vi "SNTP Light RT Driver VI_SNTP Part.vi"(7 "Configuration":T1={"Server IP Address"="206.246.122.250", "UDP Port"=123, "Synchronization Interval"=60.0, "Synchronization Threshold"=0.01, "Debug Output Strings"=TRUE, "Maximum Offset To Apply"=0.0}, 8 "error in (no error)":errorcluster, 9 "Inputs In":dbl[](array[numeric]), 11 "Outputs In":dbl[](array[numeric])) -> (0 "error out":errorcluster, 3 "Outputs Out":dbl[](array[numeric]))   [LabVIEW 2013, in "SNTP Light Custom Device Engine.lvlib"]
uses:
  SNTP Light Custom Device Engine.lvlib
  RT_Configuration_Data.ctl
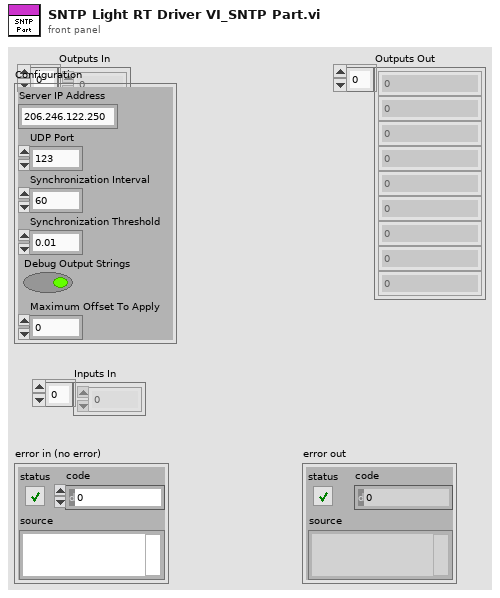
[diagram p1: front panel]
types:
  T1 = typedef "SNTP Light Custom Device Engine.lvlib/RT_Configuration_Data.ctl" = cluster{"Server IP Address":string, "UDP Port":u16, "Synchronization Interval":dbl, "Synchronization Threshold":dbl, "Debug Output Strings":bool, "Maximum Offset To Apply":dbl}
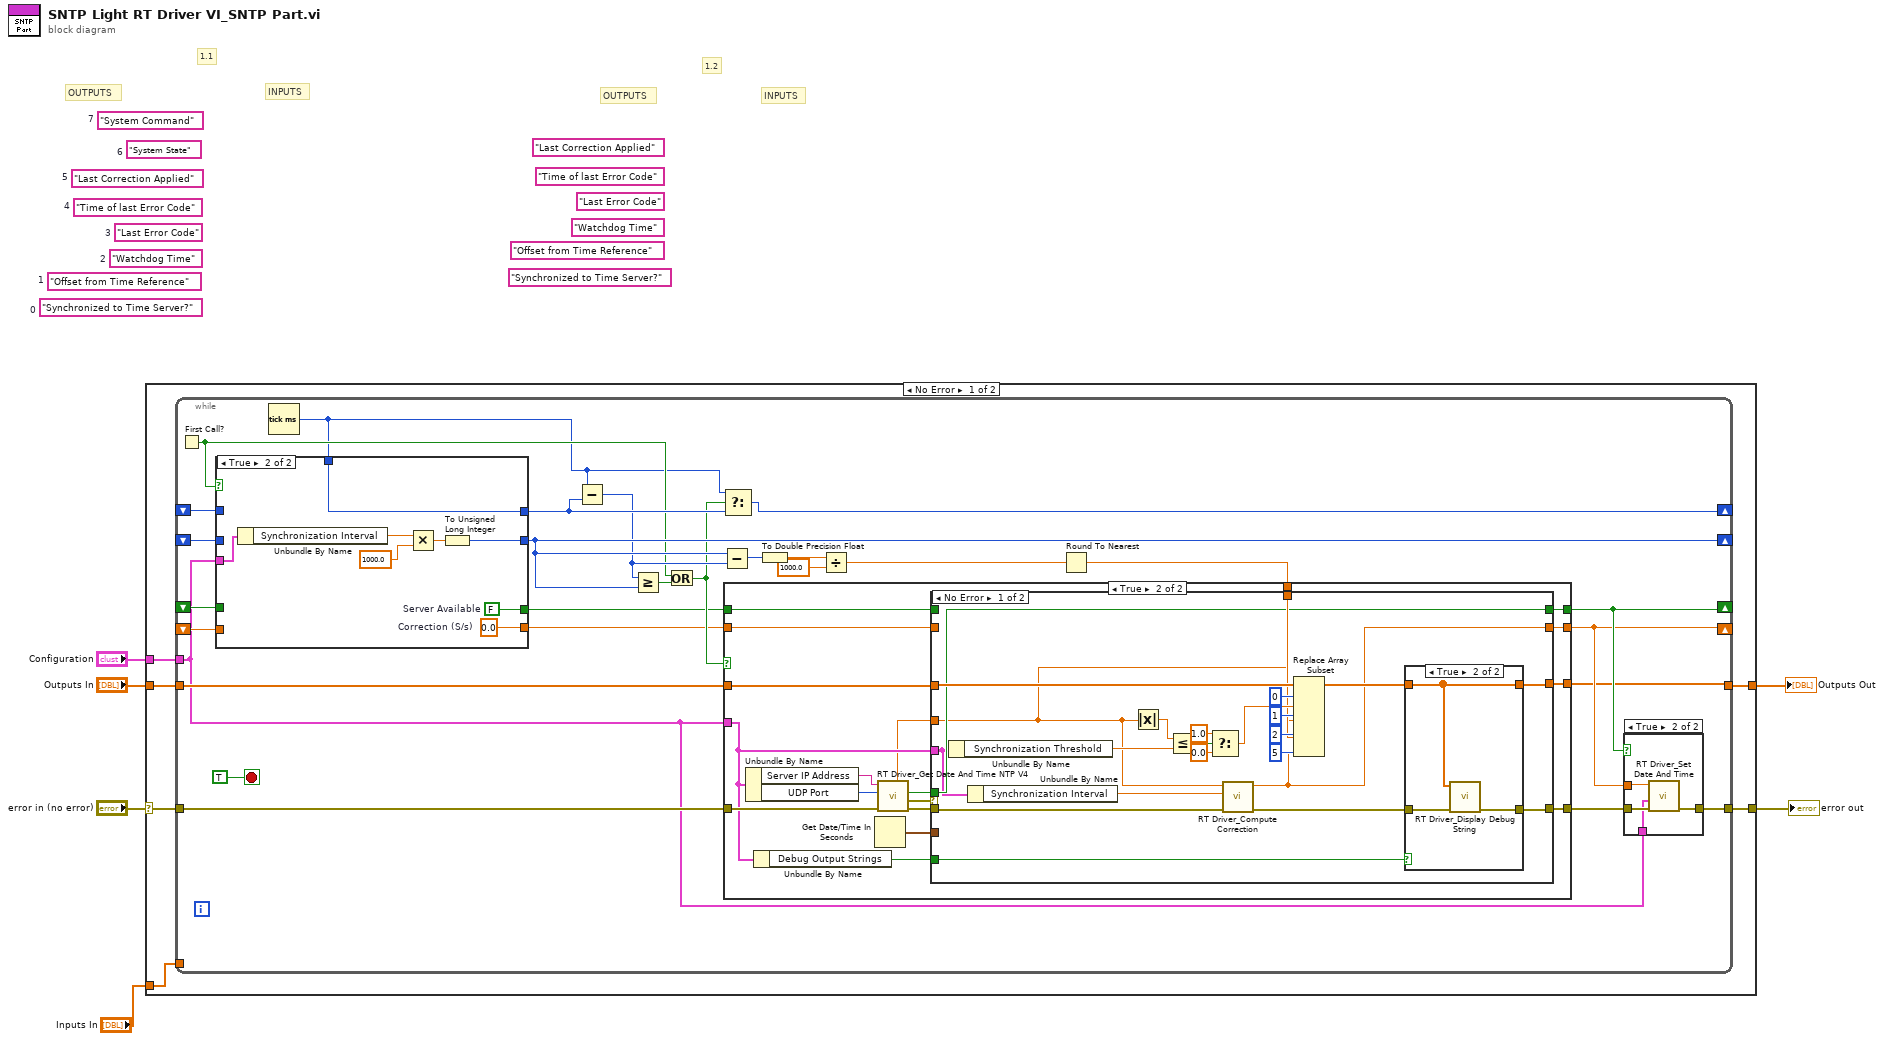
[diagram p0: block diagram]
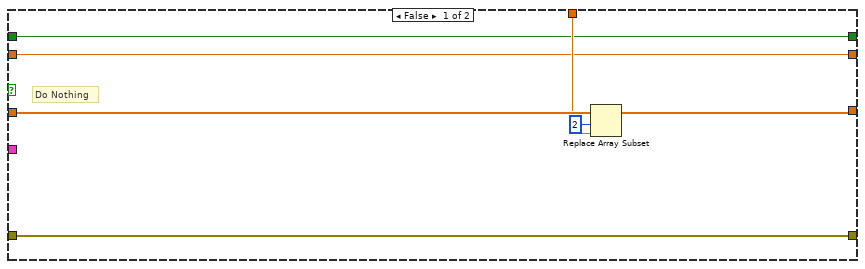
[diagram p3: hidden frame]
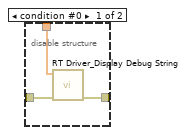
[diagram p5: hidden frame]
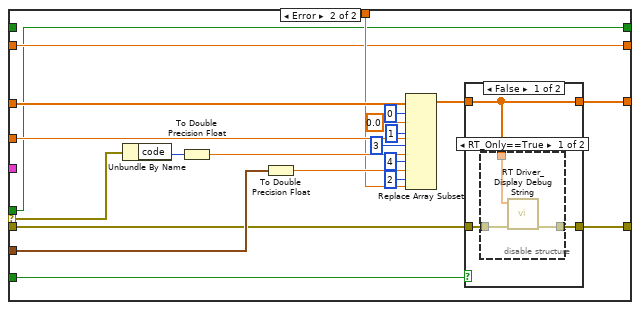
[diagram p6: hidden frame]
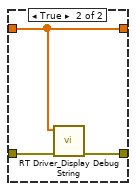
[diagram p8: hidden frame]
diagram:
  (unwired) "Last Correction Applied" ("Channel Name")
  (unwired) "Time of last Error Code" ("Channel Name")
  (unwired) "Last Error Code" ("Channel Name")
  (unwired) "Watchdog Time" ("Channel Name")
  (unwired) "Offset from Time Reference" ("Channel Name")
  (unwired) "Synchronized to Time Server?" ("Channel Name")
  (unwired) "System Command"  # 7
  (unwired) "System State"  # 6
  (unwired) "Last Correction Applied"  # 5
  (unwired) "Time of last Error Code"  # 4
  (unwired) "Last Error Code"  # 3
  (unwired) "Watchdog Time"  # 2
  (unwired) "Offset from Time Reference"  # 1
  (unwired) "Synchronized to Time Server?"  # 0
  # "INPUTS"
  # "OUTPUTS"
  # "1.1"
  # "1.2"
  # "INPUTS"
  # "OUTPUTS"
  n1 = case shown="No Error" "error in (no error)" {
    selector: "error in (no error)" -> [w10 w148]
    tunnel: [w11 w147] -> w6
    tunnel: "Outputs In" -> [w12 w147]
    tunnel: [w9 w148] -> w3
    tunnel: "Configuration" -> [w8 _]
    tunnel: "Inputs In" -> [w7 _]
    frame No Error {
      n2 = while {
        tunnel: w12 -> [w28]
        tunnel: [w14] -> w11
        tunnel: w10 -> [w27]
        tunnel: [w15] -> w9
        shift-right: [w35] -> _
        shift-left: _ -> [w39]
        tunnel: w8 -> [w13]
        shift-right: [w34] -> _
        shift-left: _ -> [w38]
        shift-right: [w20] -> _
        shift-left: _ -> [w23]
        shift-right: [w19] -> _
        shift-left: _ -> [w22]
        tunnel: w7 -> [_]
        stop <- TRUE stop-if-true
        n3 = First Call?() -> (First Call?: T/F=w18:bool)
        n4 = Tick Count (ms)() -> (millisecond timer value=w17:u32)
        n5 = case shown="True" w18 {
          tunnel: [w138 w139] -> w36
          tunnel: w39 -> [w138 _]
          tunnel: w13 -> [_ w146]
          tunnel: [w137 w142] -> w34
          tunnel: w38 -> [w137 _]
          tunnel: [w136 w141] -> w25
          tunnel: [w135 w140] -> w24
          tunnel: w23 -> [w136 _]
          tunnel: w22 -> [w135 _]
          tunnel: w17 -> [_ w139]
          frame False {
          }
          frame True {
            w140 = 0.0  # Correction (S/s)
            w141 = FALSE  # Server Available
            n6 = Unbundle By Name(w146) -> ("Synchronization Interval"=w145:dbl)
            n7 = Multiply(x=w145, y=1000.0) -> (x*y=w143:dbl)
            n8 = To Unsigned Long Integer(number=w143) -> (unsigned 32bit integer=w142:u32)
          }
        }
        n9 = Subtract(x=w17, y=w36) -> (x-y=w33:u32)
        n10 = Greater Or Equal?(x=w33, y=w34) -> (x >= y?=w37:bool)
        n11 = Or(x=w18, y=w37) -> (x .or. y?=w29:bool)
        n12 = Subtract(x=w34, y=w33) -> (x-y=w32:u32)
        n13 = Select(t=w17, s=w29, f=w36) -> (s? t:f=w35:u32)
        n14 = To Double Precision Float(number=w32) -> (double precision float=w31:dbl)
        n15 = Divide(x=w31, y=1000.0 ("x-y")) -> (x/y=w26:dbl)
        n16 = Round To Nearest(number=w26) -> (nearest integer value=w16:dbl)
        n17 = case shown="True" w29 {
          tunnel: w28 -> [w51 w65]
          tunnel: [w50 w64] -> w14
          tunnel: w27 -> [w52 w70]
          tunnel: [w52 w66] -> w21
          tunnel: w13 -> [_ w62]
          tunnel: w16 -> [w49 w60]
          tunnel: w25 -> [w46 w58]
          tunnel: w24 -> [w47 w57]
          tunnel: [w47 w56] -> w19
          tunnel: [w46 w54] -> w20
          frame False {
            # "Do Nothing"
            n18 = Replace Array Subset(array=w51, new element=w49, index=2) -> (w50:dbl[])
          }
          frame True {
            n19 = Unbundle By Name(w62) -> ("Server IP Address"=w69:string, "UDP Port"=w68:u16)
            n20 = Unbundle By Name(w62) -> ("Debug Output Strings"=w61:bool)
            n21 = Get Date/Time In Seconds() -> (seconds since 1Jan1904=w63:timestamp)
            n22 = call "RT Driver_Get Date And Time NTP V4.vi"("error in (no error) 2"=w70, "port or service name"=w68, "Timer Server IP Address"=w69) -> ("error out"=w67:errorcluster, "Last error"=w59:errorcluster, "Server Reached"=w55:bool, "Offset (s)"=w53:dbl)  [unwired: 4 in, 1 out]
            n23 = case shown="No Error" w59 {
              selector: w59 -> [_ w118]
              tunnel: w67 -> [w71 w109]
              tunnel: w53 -> [w72 w120]
              tunnel: [w80 w108] -> w66
              tunnel: w65 -> [w91 w124]
              tunnel: [w81 w106] -> w64
              tunnel: w62 -> [w78 _]
              tunnel: w63 -> [_ w113]
              tunnel: w61 -> [w85 w110]
              tunnel: w60 -> [w82 w111]
              tunnel: w58 -> [_ _]
              tunnel: w57 -> [_ w105]
              tunnel: [w74 w105] -> w56
              tunnel: w55 -> [w79 w104]
              tunnel: [w79 w104] -> w54
              frame No Error {
                n24 = Unbundle By Name(w78) -> ("Synchronization Threshold"=w92:dbl)
                n25 = Unbundle By Name(w78) -> ("Synchronization Interval"=w76:dbl)
                n26 = Absolute Value(x=w72) -> (abs(x)=w93:dbl)
                n27 = Less Or Equal?(x=w93, y=w92) -> (x <= y?=w73:bool)
                n28 = Select(t=1.0, s=w73, f=0.0) -> (s? t:f=w89:dbl)
                n29 = call "RT Driver_Compute Correction.vi"("error in (no error)"=w71, "Synchronization Interval"=w76, "Offset (s)"=w72) -> ("error out"=w77:errorcluster, "Correction (S/s)"=w74:dbl)  [unwired: 7 in]
                n30 = Replace Array Subset(array=w91, new element #1=w89, index #1=0 ("index"), new element #2=w72, index #2=1 ("index"), new element #3=w82, index #3=2 ("index"), new element #4=w74, index #4=5 ("index")) -> (w84:dbl[])
                n31 = case shown="True" w85 {
                  tunnel: w77 -> [w96 w103]
                  tunnel: w84 -> [w94 w101]
                  tunnel: [w94 w101] -> w81
                  tunnel: [w95 w102] -> w80
                  frame False {
                    n32 = disable-structure shown="RT_Only==False, Default" {
                      disable-tunnel: w96 -> [w99 w100]
                      disable-tunnel: [w98 w100] -> w95
                      disable-tunnel: w94 -> [w97 _]
                      frame condition #0 {
                        n33 = call "RT Driver_Display Debug String.vi"("error in (no error)"=w99, "Outputs In"=w97) -> ("error out"=w98:errorcluster)  [unwired: 9 in]
                      }
                      frame condition #1 (active) {
                      }
                    }
                  }
                  frame True {
                    n34 = call "RT Driver_Display Debug String.vi"("error in (no error)"=w103, "Outputs In"=w101) -> ("error out"=w102:errorcluster)  [unwired: 9 in]
                  }
                }
              }
              frame Error {
                n35 = Unbundle By Name(w118) -> ("code"=w117:i32)
                n36 = To Double Precision Float(number=w117) -> (double precision float=w116:dbl)
                n37 = To Double Precision Float(number=w113) -> (double precision float=w114:dbl)
                n38 = Replace Array Subset(array=w124, new element #1=0.0 ("new element/subarray"), index #1=0 ("index"), new element #2=w120, index #2=1 ("index"), new element #3=w116, index #3=3 ("index"), new element #4=w114, index #4=4 ("index"), new element #5=w111, index #5=2 ("index")) -> (w107:dbl[])
                n39 = case shown="False" w110 {
                  tunnel: w109 -> [w127 w133]
                  tunnel: w107 -> [w125 w132]
                  tunnel: [w125 w132] -> w106
                  tunnel: [w126 w134] -> w108
                  frame False {
                    n40 = disable-structure shown="RT_Only==True" {
                      disable-tunnel: w127 -> [w130 w131]
                      disable-tunnel: [w129 w131] -> w126
                      disable-tunnel: w125 -> [w128 _]
                      frame condition #0 {
                        n41 = call "RT Driver_Display Debug String.vi"("error in (no error)"=w130, "Outputs In"=w128) -> ("error out"=w129:errorcluster)  [unwired: 9 in]
                      }
                      frame condition #1 (active) {
                      }
                    }
                  }
                  frame True {
                    n42 = call "RT Driver_Display Debug String.vi"("error in (no error)"=w133, "Outputs In"=w132) -> ("error out"=w134:errorcluster)  [unwired: 9 in]
                  }
                }
              }
            }
          }
        }
        n43 = case shown="True" w20 {
          tunnel: w21 -> [w41 w45]
          tunnel: [w41 w44] -> w15
          tunnel: w19 -> [_ w43]
          tunnel: w13 -> [_ w42]
          frame False {
          }
          frame True {
            n44 = call "RT Driver_Set Date And Time.vi"("error in (no error)"=w45, "Configuration"=w42, "Correction (S/s)"=w43) -> ("error out"=w44:errorcluster)  [unwired: 8 in]
          }
        }
      }
    }
    frame Error {
    }
  }
  "Outputs Out" <- w6
  "error out" <- w3
